vi "DCC_get_curr_lmt_state.vi"(8 "Error In":errorcluster, 10 "Module No":i16, 11 "DLL Path":path) -> (0 "Error Out":errorcluster, 2 "Module No":i16, 3 "DLL Path":path, 4 "LMT State":i16)   [LabVIEW 2017]
doc: "The procedure is used to check whether the current limit is reached ( for cooling device on Connector 3) on the DCC module ‘mod_no’.\n\nThe ‘state’ variable is set to 0 or 1 according to the Current limit flag.\n\nAugust 2018\nFrank Quadt & Stefan Smietana\ninfo@becker-hickl.com"
panel:
  # "(c) 2021 Becker & Hickl GmbH\n     All Rights Reserved."
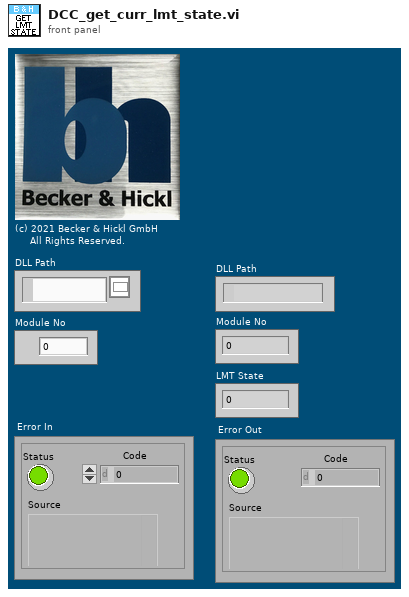
[diagram p1: front panel]
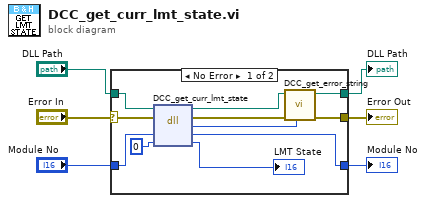
[diagram p0: block diagram]
diagram:
  n1 = case shown="No Error" "Error In" {
    selector: "Error In" -> [w17 w18]
    tunnel: [w8 w18] -> w5
    tunnel: [w10 w20] -> w4
    tunnel: "DLL Path" -> [w15 w20]
    tunnel: "Module No" -> [w14 w19]
    tunnel: [w13 w19] -> w1
    frame No Error {
      n2 = dll-call lib="C:/Program Files/BH/DCC/DLL/dcc32.dll" fn="DCC_get_curr_lmt_state"(path in=w15, error in=w17, "ModuleNo"=w14, "State"=i16 0) -> (path out=w16:path, error out=w9:errorcluster, "return type"=w7:i16, "ModuleNo"=w13:i16, "State"=→"LMT State":i16)  [unwired: 1 in]
      n3 = call "DCC_get_error_string.vi"("Error ID"=w7, "Error In"=w9, "DLL Path"=w16) -> ("Error Out"=w8:errorcluster, "DLL Path"=w10:path)  [unwired: 6 in, 1 out]
    }
    frame Error {
    }
  }
  "Error Out" <- w5
  "DLL Path" <- w4
  "Module No" <- w1
